vi "test-SwerveDrvPoseEst2-testFollowTrajectory.vi"(0 "chassisSpeedsGenerator":refnum<vi>, 1 "TRAJECTORY":T12 {"States"."POSE"."ROTATION"."SIN" format="%13.4f"; "States"."POSE"."ROTATION"."COS" format="%13.4f"; "States"."POSE"."ROTATION"."VALUE" format="%13.4f"; "States"."POSE"."TRANSLATION"."Y" format="%14.3f"; "States"."POSE"."TRANSLATION"."X" format="%14.3f"; "TotalTImeSecs" format="%20.3f"}, 2 "SwerveDrivePoseEstimate2":T5={"M_Vision_K"=[], "m_nominal_dT"=0.0, "m_PrevTime_Sec"=0.0, "Pose_Buffer"={"TimeStamps"=[], "DataArray"=[], "Min_TimeStamp"=0.0, "Max_TimeStamp"=0.0, "ItemCount"=0, "MaxBufferTime"=0.0}, "Swerve_Drive_Kinematics"={"NumModules"=0, "InverseKinematics"=[], "ForwardKinematics"=[], "Modules"=[], "PrevCoR"={"X"=0.0, "Y"=0.0}, "SavedModuleStates"=[]}, "Swerve_Drive_Odom"={"POSE"={"TRANSLATION"={"X"=0.0, "Y"=0.0}, "ROTATION"={"VALUE"=0.0, "COS"=0.0, "SIN"=0.0}}, "GyroOffset"={"VALUE"=0.0, "COS"=0.0, "SIN"=0.0}, "PreviousAngle"={"VALUE"=0.0, "COS"=0.0, "SIN"=0.0}, "PrevModulePositions"=[], "NumModules"=0}, "M_Q"=[], "NumModules"=-1} {"Swerve_Drive_Odom"."PrevModulePositions"."Angle"."SIN" format="%13.4f"; "Swerve_Drive_Odom"."PrevModulePositions"."Angle"."COS" format="%13.4f"; "Swerve_Drive_Odom"."PrevModulePositions"."Angle"."VALUE" format="%13.4f"; "Swerve_Drive_Odom"."PreviousAngle"."SIN" format="%13.4f"; "Swerve_Drive_Odom"."PreviousAngle"."COS" format="%13.4f"; "Swerve_Drive_Odom"."PreviousAngle"."VALUE" format="%13.4f"; "Swerve_Drive_Odom"."GyroOffset"."SIN" format="%13.4f"; "Swerve_Drive_Odom"."GyroOffset"."COS" format="%13.4f"; "Swerve_Drive_Odom"."GyroOffset"."VALUE" format="%13.4f"; "Swerve_Drive_Odom"."POSE"."ROTATION"."SIN" format="%13.4f"; "Swerve_Drive_Odom"."POSE"."ROTATION"."COS" format="%13.4f"; "Swerve_Drive_Odom"."POSE"."ROTATION"."VALUE" format="%13.4f"; "Swerve_Drive_Odom"."POSE"."TRANSLATION"."Y" format="%14.3f"; "Swerve_Drive_Odom"."POSE"."TRANSLATION"."X" format="%14.3f"; "Swerve_Drive_Kinematics"."SavedModuleStates"."Angle"."SIN" format="%13.4f"; "Swerve_Drive_Kinematics"."SavedModuleStates"."Angle"."COS" format="%13.4f"; "Swerve_Drive_Kinematics"."SavedModuleStates"."Angle"."VALUE" format="%13.4f"; "Swerve_Drive_Kinematics"."PrevCoR"."Y" format="%14.3f"; "Swerve_Drive_Kinematics"."PrevCoR"."X" format="%14.3f"; "Swerve_Drive_Kinematics"."Modules"."Y" format="%14.3f"; "Swerve_Drive_Kinematics"."Modules"."X" format="%14.3f"}, 5 "genVisionMeasurement":refnum<vi>, 7 "StartingPose":T2={"TRANSLATION"={"X"=0.0, "Y"=0.0}, "ROTATION"={"VALUE"=0.0, "COS"=1.0, "SIN"=0.0}} {"ROTATION"."SIN" format="%13.4f"; "ROTATION"."COS" format="%13.4f"; "ROTATION"."VALUE" format="%13.4f"; "TRANSLATION"."Y" format="%14.3f"; "TRANSLATION"."X" format="%14.3f"}, 9 "EndingPose":T2={"TRANSLATION"={"X"=0.0, "Y"=0.0}, "ROTATION"={"VALUE"=0.0, "COS"=1.0, "SIN"=0.0}} {"ROTATION"."SIN" format="%13.4f"; "ROTATION"."COS" format="%13.4f"; "ROTATION"."VALUE" format="%13.4f"; "TRANSLATION"."Y" format="%14.3f"; "TRANSLATION"."X" format="%14.3f"}, 11 "dt_Seconds":dbl, 12 "VisionUpdateRate":dbl, 13 "VisionUpdateDelay":dbl, 14 "CheckError":bool) -> (4 "Test Passed":bool, 6 "Output Data":T1, 15 "DataForGraph":cluster{dbl[], dbl[]}[](array[cluster]))   [LabVIEW 2019]
uses:
  <vilib>/Rock Robotics/WPI/ThirdParty/JAS_Junk/TrajLib/Trajectory_Library.lvlib
  <vilib>/Rock Robotics/WPI/ThirdParty/JAS_Junk/TrajLib/TypeDef/TRANSLATION2D.ctl
  <vilib>/Rock Robotics/WPI/ThirdParty/JAS_Junk/TrajLib/TypeDef/ROTATION2D.ctl
  <vilib>/Rock Robotics/WPI/ThirdParty/JAS_Junk/TrajLib/TypeDef/POSE2D.ctl
  <vilib>/Rock Robotics/WPI/ThirdParty/JAS_Junk/TrajLib/TypeDef/TRAJ_STATE.ctl
  <vilib>/Rock Robotics/WPI/ThirdParty/JAS_Junk/TrajLib/TypeDef/TRAJECTORY.ctl
  <vilib>/Analysis/Matrix/Datatypes/RealMatrix.ctl
  <vilib>/Analysis/Matrix/NI_Matrix.lvlib
  <vilib>/Rock Robotics/WPI/ThirdParty/JAS_Junk/TrajLib/TypeDef/TIME_INTERPOLATABLE_VARIANT.ctl
  <vilib>/Rock Robotics/WPI/ThirdParty/JAS_Junk/TrajLib/TypeDef/SWERVE_DRIVE_MODULE_STATE.ctl
  <vilib>/Rock Robotics/WPI/ThirdParty/JAS_Junk/TrajLib/TypeDef/SWERVE_DRIVE_KINEMATICS.ctl
  <vilib>/Rock Robotics/WPI/ThirdParty/JAS_Junk/TrajLib/TypeDef/SWERVE_DRIVE_MODULE_POSITION.ctl
  <vilib>/Rock Robotics/WPI/ThirdParty/JAS_Junk/TrajLib/TypeDef/SWERVE_DRIVE_ODOMETRY.ctl
  <vilib>/Rock Robotics/WPI/ThirdParty/JAS_Junk/TrajLib/TypeDef/SWERVE_DRIVE_POSE_EST2.ctl
panel:
  in  "UseVIsion":bool=TRUE
  out "error out":errorcluster
  in  "error in (no error)":errorcluster
  # "<3, 1>"
  # "<3, 3>"
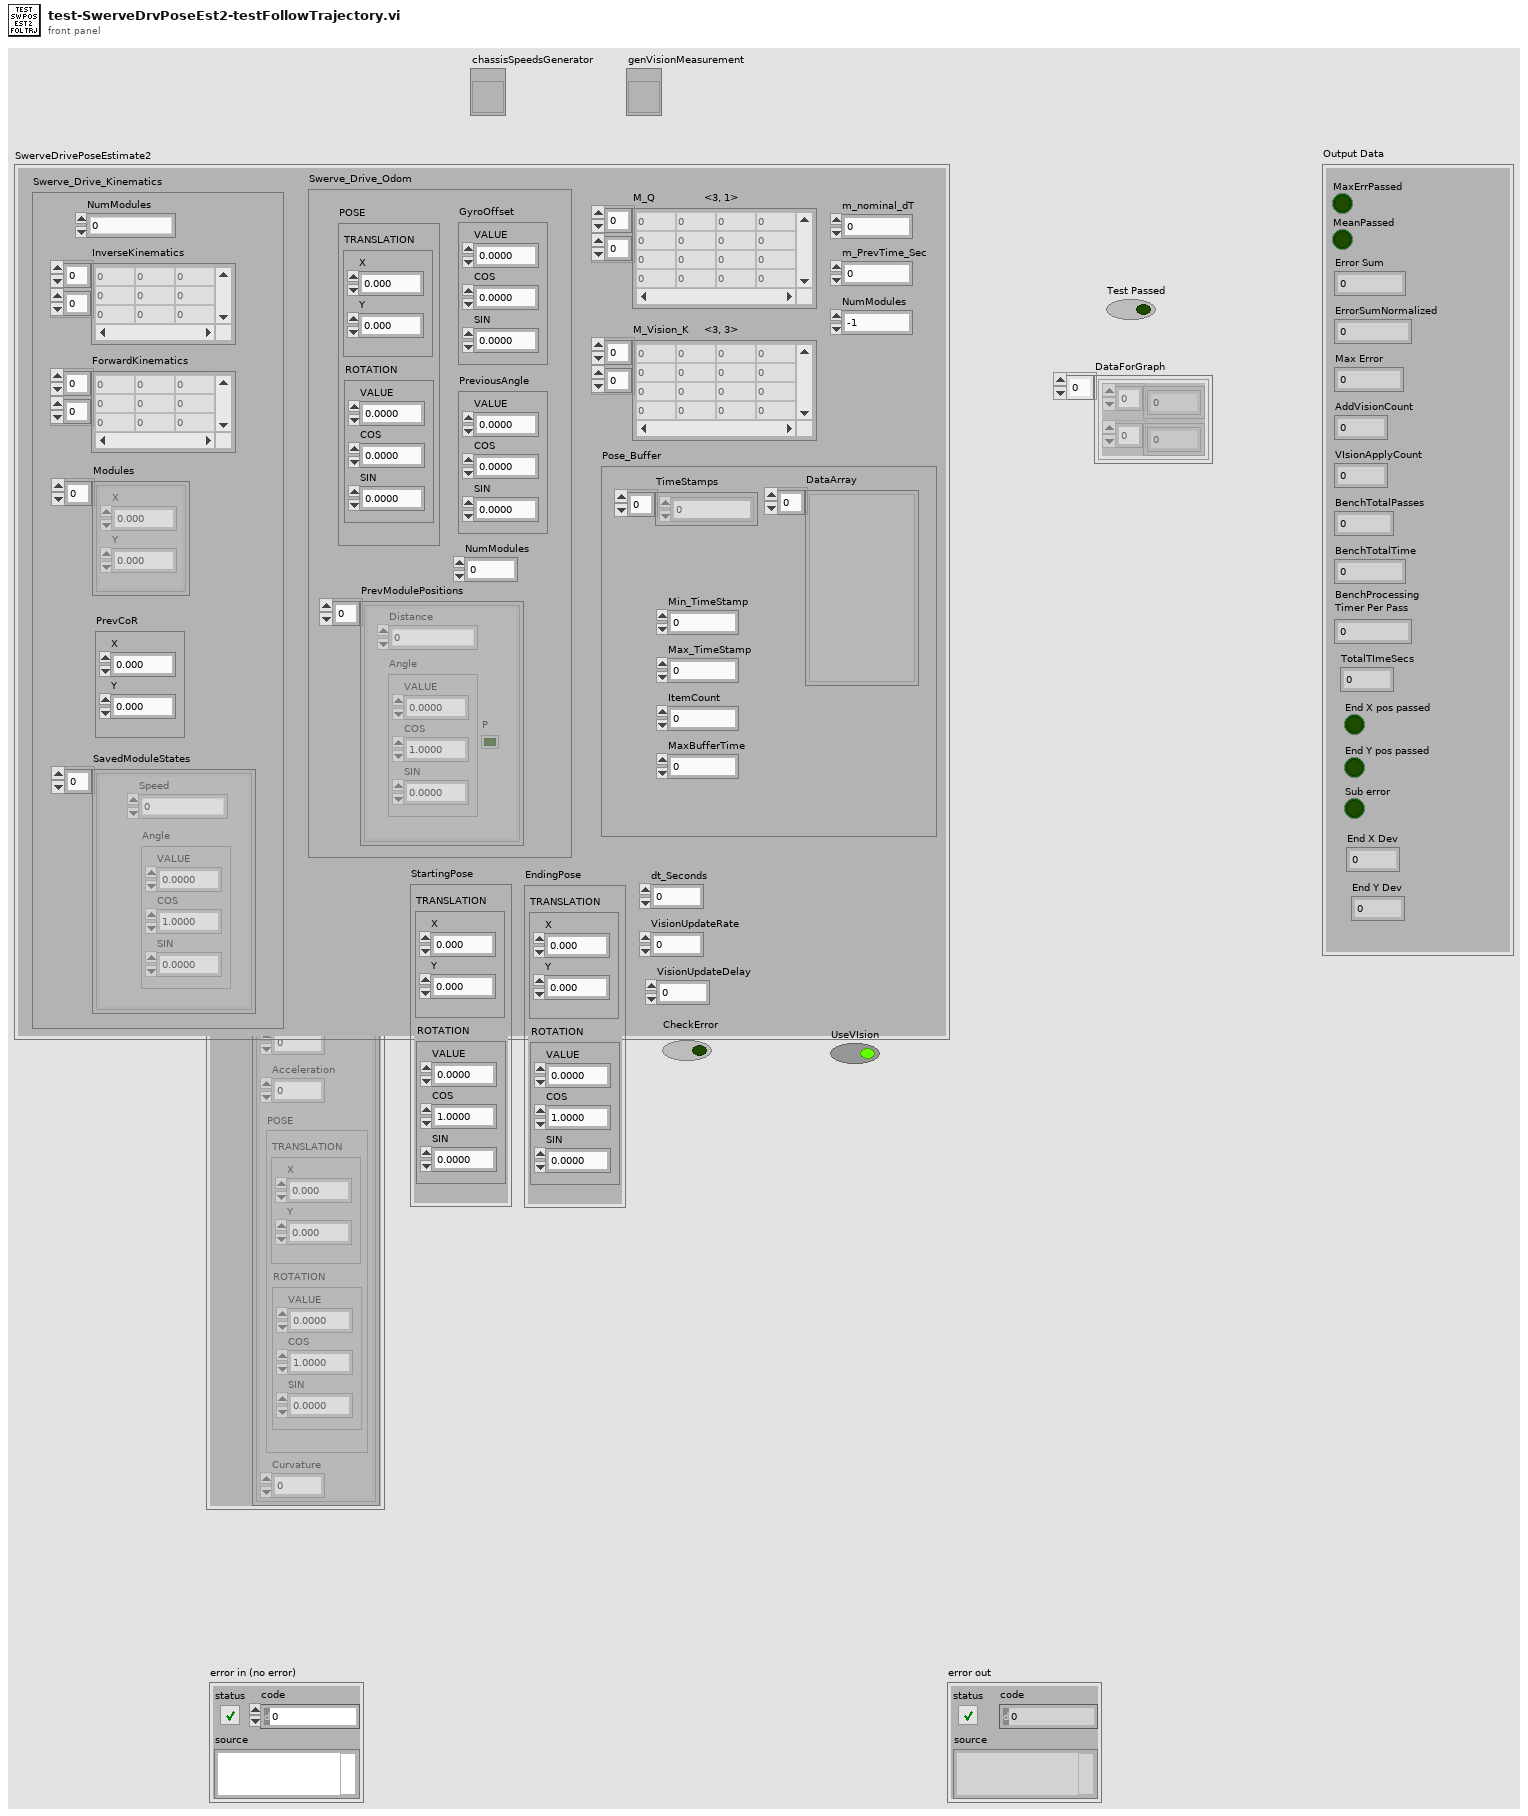
[diagram p1: front panel]
types:
  T1 = cluster{"MaxErrPassed":bool, "MeanPassed":bool, "Error Sum":dbl, "ErrorSumNormalized":dbl, "Max Error":dbl, "AddVisionCount":i32, "VIsionApplyCount":i32, "BenchTotalPasses":dbl, "BenchTotalTime":dbl, "BenchProcessing \nTimer Per Pass":dbl, "TotalTImeSecs":dbl, "End X pos passed":bool, "End Y pos passed":bool, "Sub error":bool, "End X Dev":dbl, "End Y Dev":dbl}
  T2 = typedef "Trajectory_Library.lvlib/POSE2D.ctl" = cluster{"TRANSLATION":T3, "ROTATION":T4}
  T3 = typedef "Trajectory_Library.lvlib/TRANSLATION2D.ctl" = cluster{"X":dbl, "Y":dbl}
  T4 = typedef "Trajectory_Library.lvlib/ROTATION2D.ctl" = cluster{"VALUE":dbl, "COS":dbl, "SIN":dbl}
  T5 = typedef "Trajectory_Library.lvlib/SWERVE_DRIVE_POSE_EST2.ctl" = cluster{"M_Vision_K":T6, "m_nominal_dT":dbl, "m_PrevTime_Sec":dbl, "Pose_Buffer":T7, "Swerve_Drive_Kinematics":T8, "Swerve_Drive_Odom":T10, "M_Q":T6, "NumModules":i32}
  T6 = typedef "NI_Matrix.lvlib/RealMatrix.ctl" = dbl[][]
  T7 = typedef "Trajectory_Library.lvlib/TIME_INTERPOLATABLE_VARIANT.ctl" = cluster{"TimeStamps":dbl[], "DataArray":variant[], "Min_TimeStamp":dbl, "Max_TimeStamp":dbl, "ItemCount":i32, "MaxBufferTime":dbl}
  T8 = typedef "Trajectory_Library.lvlib/SWERVE_DRIVE_KINEMATICS.ctl" = cluster{"NumModules":i32, "InverseKinematics":T6, "ForwardKinematics":T6, "Modules":T3[], "PrevCoR":T3, "SavedModuleStates":T9[]}
  T9 = typedef "Trajectory_Library.lvlib/SWERVE_DRIVE_MODULE_STATE.ctl" = cluster{"Speed":dbl, "Angle":T4}
  T10 = typedef "Trajectory_Library.lvlib/SWERVE_DRIVE_ODOMETRY.ctl" = cluster{"POSE":T2, "GyroOffset":T4, "PreviousAngle":T4, "PrevModulePositions":T11[], "NumModules":i32}
  T11 = typedef "Trajectory_Library.lvlib/SWERVE_DRIVE_MODULE_POSITION.ctl" = cluster{"Distance":dbl, "Angle":T4, "P":bool}
  T12 = typedef "Trajectory_Library.lvlib/TRAJECTORY.ctl" = cluster{"TotalTImeSecs":dbl, "States":T13[]}
  T13 = typedef "Trajectory_Library.lvlib/TRAJ_STATE.ctl" = cluster{"TimeSeconds":dbl, "Velocity":dbl, "Acceleration":dbl, "POSE":T2, "Curvature":dbl}
  T14 = typedef "Trajectory_Library.lvlib/TIME_INTERPOLATABLE_POSE2D.ctl" = cluster{"TimeStamps":dbl[], "Pose":T2[], "Min_TimeStamp":dbl, "Max_TimeStamp":dbl, "ItemCount":i32, "MaxBufferTime":dbl}
  T15 = typedef "Trajectory_Library.lvlib/TRANSFORM2D.ctl" = cluster{"TRANSLATION":T3, "ROTATION":T4, "xF":bool}
  T16 = typedef "Trajectory_Library.lvlib/CHASSIS_SPEEDS.ctl" = cluster{"vX":dbl, "vY":dbl, "vOmega":dbl}
  T17 = cluster{bool, bool, "Error Sum":dbl, dbl, dbl, i32, i32, "TotalPasses":dbl, "TotalTime":dbl, dbl, "TotalTImeSecs":dbl, bool, bool, bool, dbl, dbl}
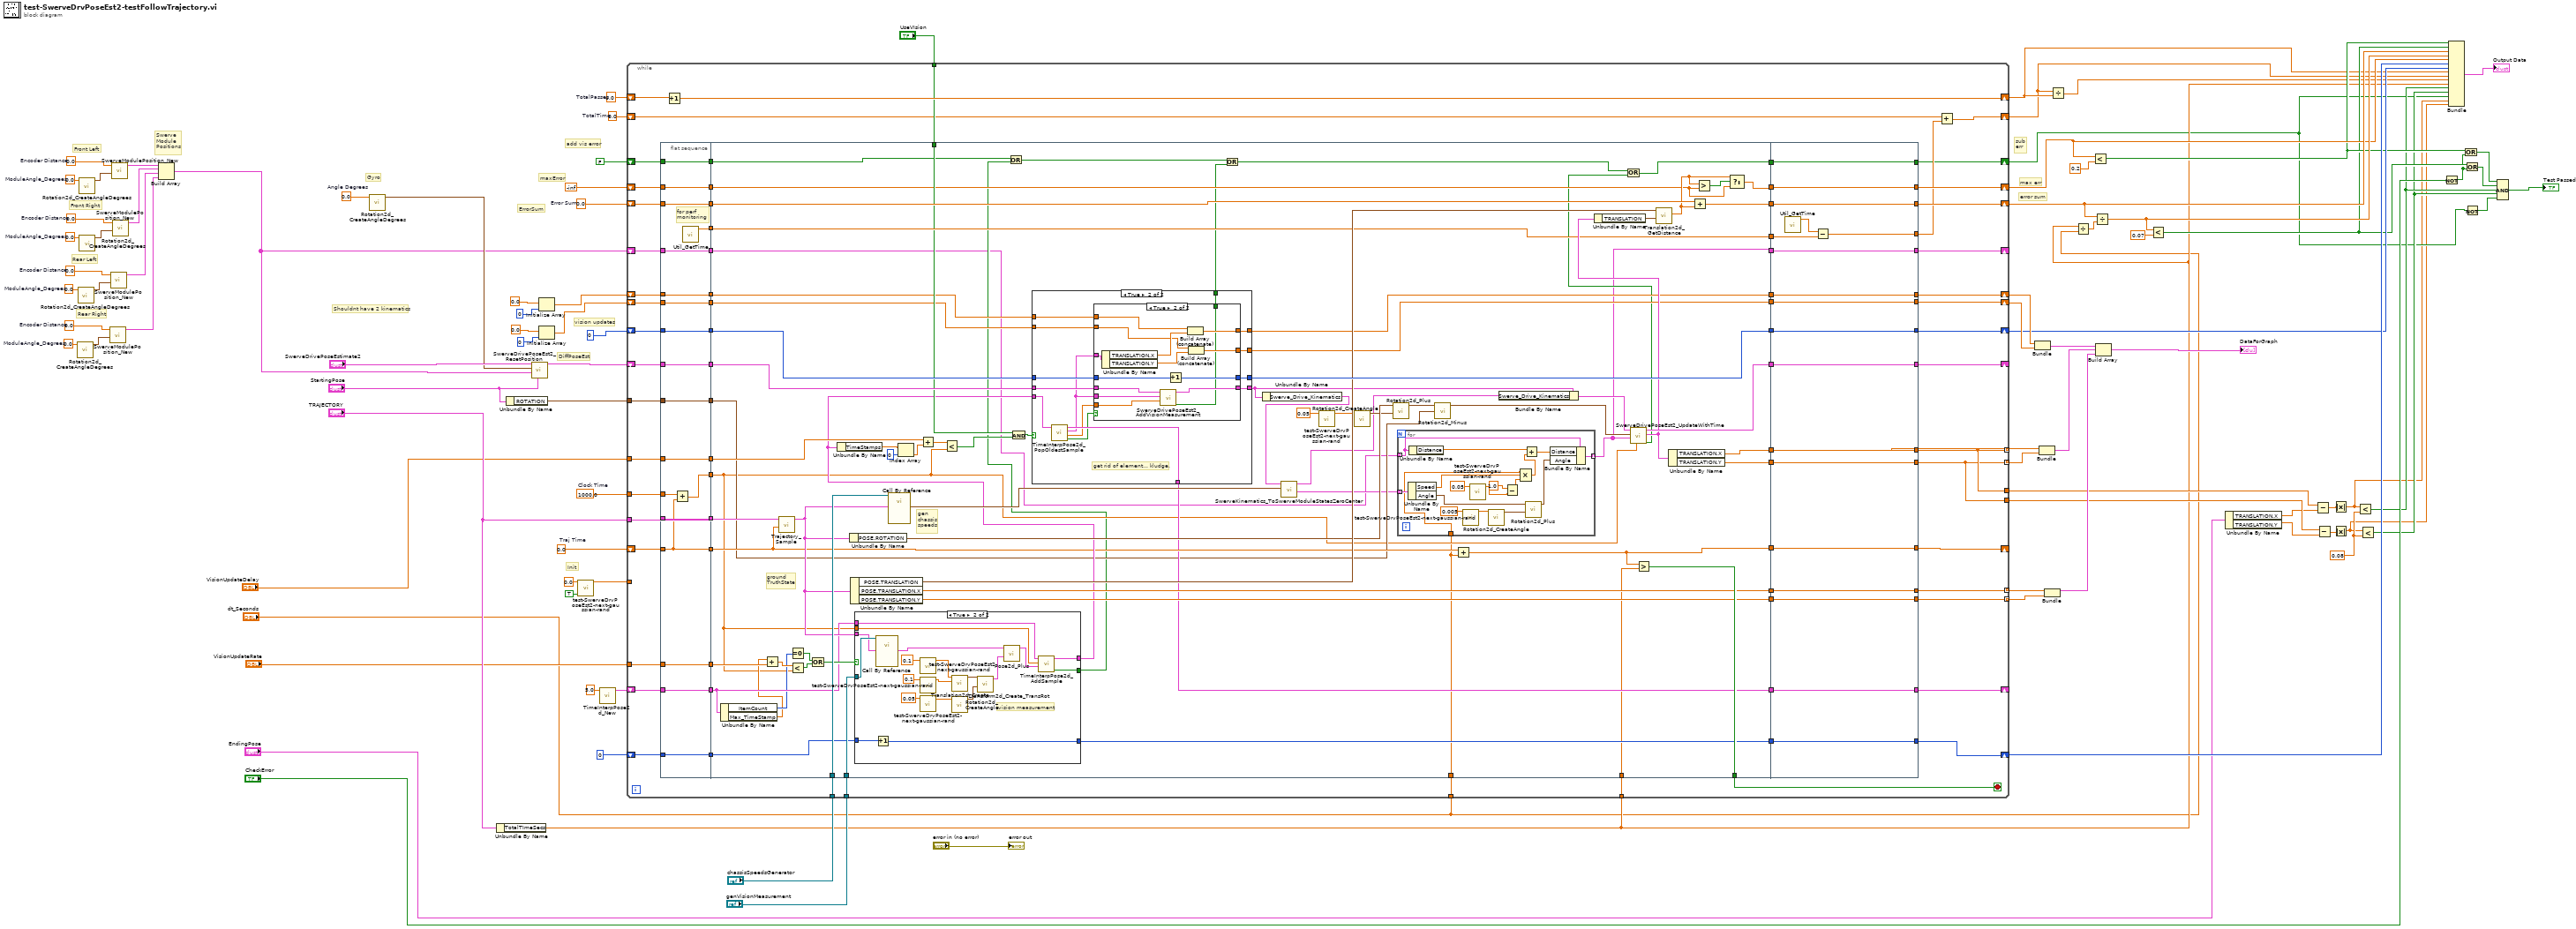
[diagram p0: block diagram]
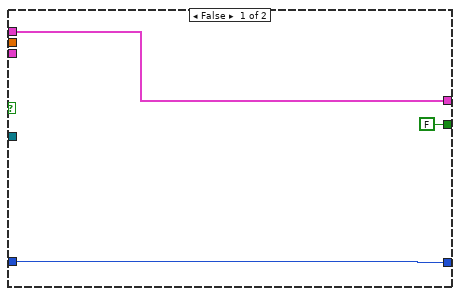
[diagram p2: hidden frame]
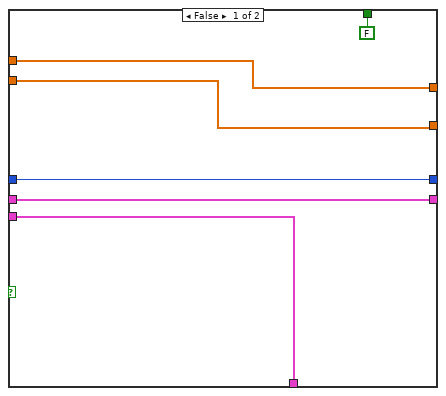
[diagram p3: hidden frame]
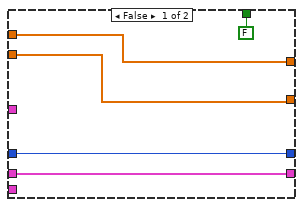
[diagram p4: hidden frame]
diagram:
  w14 = 0.0  # ModuleAngle_Degrees
  w12 = 0.0  # Encoder Distance
  w11 = 0.0  # ModuleAngle_Degrees
  w9 = 0.0  # Encoder Distance
  w8 = 0.0  # ModuleAngle_Degrees
  w6 = 0.0  # Encoder Distance
  w4 = 0.0  # ModuleAngle_Degrees
  w2 = 0.0  # Encoder Distance
  w39 = 0.08
  w64 = 1000.0  # Clock Time
  w72 = 0.0  # Angle Degrees
  w92 = 0.0  # TotalPasses
  w91 = 0.0  # TotalTime
  w86 = 0.0  # Error Sum
  w76 = 0.0  # Traj Time
  # "Shouldnt have 2 kinematics"
  # "Front Left"
  # "Swerve\nModule\nPositions"
  # "Rear Right"
  # "Rear Left"
  # "Front Right"
  # "Init"
  # "sub\nerr"
  # "add vis error"
  # "max err"
  # "error sum"
  # "Gyro"
  # "ErrorSum"
  # "maxError"
  # "vision updates"
  # "DiffPoseEst"
  n1 = call <vilib>:"Rotation2d_CreateAngleDegrees.vi"("Angle_Degrees"=w14) -> ("ROTATION"=w13:T4)  [unwired: 10 in]
  n2 = call <vilib>:"Rotation2d_CreateAngleDegrees.vi"("Angle_Degrees"=w11) -> ("ROTATION"=w10:T4)  [unwired: 10 in]
  n3 = call <vilib>:"Rotation2d_CreateAngleDegrees.vi"("Angle_Degrees"=w4) -> ("ROTATION"=w3:T4)  [unwired: 10 in]
  n4 = call <vilib>:"Rotation2d_CreateAngleDegrees.vi"("Angle_Degrees"=w8) -> ("ROTATION"=w7:T4)  [unwired: 10 in]
  n5 = call <vilib>:"SwerveModulePosition_New.vi"("ROTATION"=w13, "Distance"=w12) -> ("SWERVE_DRIVE_MODULE_POSITION"=w17:T11)  [unwired: 9 in]
  n6 = call <vilib>:"SwerveModulePosition_New.vi"("ROTATION"=w10, "Distance"=w9) -> ("SWERVE_DRIVE_MODULE_POSITION"=w16:T11)  [unwired: 9 in]
  n7 = call <vilib>:"SwerveModulePosition_New.vi"("ROTATION"=w3, "Distance"=w2) -> ("SWERVE_DRIVE_MODULE_POSITION"=w5:T11)  [unwired: 9 in]
  n8 = call <vilib>:"SwerveModulePosition_New.vi"("ROTATION"=w7, "Distance"=w6) -> ("SWERVE_DRIVE_MODULE_POSITION"=w15:T11)  [unwired: 9 in]
  n9 = Build Array(w5, w15, w16, w17) -> (w1:T11[])
  n10 = call <vilib>:"Rotation2d_CreateAngleDegrees.vi"("Angle_Degrees"=w72) -> ("ROTATION"=w71:T4)  [unwired: 10 in]
  n11 = Unbundle By Name("TRAJECTORY") -> ("TotalTImeSecs"=w29:dbl)
  n12 = Unbundle By Name("StartingPose") -> ("ROTATION"=w47:T4)
  n13 = call <vilib>:"SwerveDrivePoseEst2_ResetPosition.vi"("Pose"="StartingPose", "Module Positions"=w1, "Gyro"=w71, "in SwerveDrivePoseEst2"="SwerveDrivePoseEstimate2") -> ("Out SwerveDrivePoseEst2"=w73:T5)  [unwired: 7 in]
  n14 = Initialize Array(0.0, 0 ("dimension size")) -> (w59:dbl[])
  n15 = Initialize Array(0.0, 0 ("dimension size")) -> (w58:dbl[])
  n16 = call "test-SwerveDrvPoseEst2-next-gaussian-rand.vi"("Init"=TRUE, "Multiplier"=0.0 ("R2")) -> ("Gaussian white noise"=w18:dbl)  [unwired: 9 in]
  n17 = call <vilib>:"TimeInterpPose2d_New.vi"("MaxTime"=5.0) -> ("TimeInterpPose"=w68:T14)  [unwired: 10 in]
  n18 = while {
    shift-right: [w170] -> _
    shift-left: w76 -> [w166]
    tunnel: "TRAJECTORY" -> [w168]
    tunnel: w29 -> [w169]
    tunnel: "VisionUpdateRate" -> [w124]
    shift-right: [w135] -> _
    shift-left: w73 -> [w167]
    tunnel: [w106] -> w77 mode=indexing
    tunnel: [w105] -> w78 mode=indexing
    shift-right: [w164] -> w49
    shift-left: 0 -> [w165]
    tunnel: [w163] -> w82 mode=indexing
    tunnel: [w162] -> w83 mode=indexing
    shift-right: [w159] -> w52
    shift-left: -inf -> [w158]
    shift-right: [w160] -> w54
    shift-left: w86 -> [w161]
    shift-right: [w101] -> w31
    shift-left: w91 -> [w102]
    shift-right: [w137] -> w32
    shift-left: w92 -> [w138]
    tunnel: "UseVIsion" -> [w136]
    shift-right: [w132] -> _
    shift-left: w1 -> [w133]
    shift-right: [w127] -> _
    shift-left: w68 -> [w129]
    tunnel: "chassisSpeedsGenerator" -> [w130]
    tunnel: "genVisionMeasurement" -> [w125]
    tunnel: "VisionUpdateDelay" -> [w123]
    tunnel: w64 -> [w121]
    shift-right: [w116] -> w57
    shift-left: w59 -> [w119]
    shift-right: [w114] -> w56
    shift-left: w58 -> [w117]
    shift-right: [w110] -> w50
    shift-left: 0 -> [w111]
    tunnel: w47 -> [w107]
    tunnel: [w106] -> w45
    tunnel: [w105] -> w44
    shift-right: [w98] -> w24
    shift-left: FALSE -> [w99]
    tunnel: "dt_Seconds" -> [w96]
    tunnel: w18 -> [_]
    stop <- w157 stop-if-true
    n19 = flat-sequence {
      tunnel: w158 -> [w183]
      tunnel: w161 -> [w184]
      tunnel: w165 -> [w185]
      tunnel: w166 -> [w177]
      tunnel: w167 -> [w186]
      tunnel: w124 -> [w187]
      tunnel: w168 -> [w188]
      tunnel: [w188] -> w156
      tunnel: [w187] -> w155
      tunnel: [w186] -> w154
      tunnel: [w177] -> w153
      tunnel: [w185] -> w152
      tunnel: [w184] -> w151
      tunnel: [w183] -> w150
      tunnel: [w179] -> w140
      tunnel: [w182] -> w134
      tunnel: w133 -> [w182]
      tunnel: w129 -> [w181]
      tunnel: [w181] -> w128
      tunnel: w123 -> [w180]
      tunnel: [w180] -> w122
      tunnel: w121 -> [w178]
      tunnel: [w176] -> w120
      tunnel: w119 -> [w176]
      tunnel: [w175] -> w118
      tunnel: w117 -> [w175]
      tunnel: [w174] -> w112
      tunnel: w111 -> [w174]
      tunnel: [w173] -> w108
      tunnel: w107 -> [w173]
      tunnel: [w172] -> w104
      tunnel: [w171] -> w100
      tunnel: w99 -> [w171]
      tunnel: [w262] -> w157
      tunnel: w169 -> [w205]
      tunnel: w156 -> [w260]
      tunnel: w155 -> [w232]
      tunnel: w154 -> [w259]
      tunnel: w153 -> [w218]
      tunnel: w152 -> [w255]
      tunnel: w151 -> [w248]
      tunnel: w150 -> [w204]
      tunnel: [w261] -> w149
      tunnel: [w258] -> w148
      tunnel: [w257] -> w147
      tunnel: [w256] -> w146
      tunnel: [w254] -> w145
      tunnel: [w253] -> w144
      tunnel: [w252] -> w143
      tunnel: [w247] -> w142
      tunnel: [w244] -> w141
      tunnel: w140 -> [w243]
      tunnel: [w243] -> w139
      tunnel: w136 -> [w226]
      tunnel: w134 -> [w189]
      tunnel: [w191] -> w131
      tunnel: w130 -> [w239]
      tunnel: w128 -> [w230]
      tunnel: [w217] -> w126
      tunnel: w125 -> [w237]
      tunnel: w122 -> [w223]
      tunnel: w120 -> [w216]
      tunnel: w118 -> [w215]
      tunnel: [w214] -> w115
      tunnel: [w213] -> w113
      tunnel: w112 -> [w212]
      tunnel: [w211] -> w109
      tunnel: w108 -> [w207]
      tunnel: w104 -> [w206]
      tunnel: w100 -> [w199]
      tunnel: [w201] -> w97
      tunnel: w96 -> [w190]
      tunnel: [w350] -> w159
      tunnel: [w351] -> w160
      tunnel: [w352] -> w162
      tunnel: [w353] -> w163
      tunnel: [w354] -> w164
      tunnel: [w355] -> w105
      tunnel: [w356] -> w106
      tunnel: [w357] -> w135
      tunnel: [w358] -> w170
      tunnel: w149 -> [w358]
      tunnel: w148 -> [w357]
      tunnel: w147 -> [w356]
      tunnel: w146 -> [w355]
      tunnel: w145 -> [w354]
      tunnel: w144 -> [w353]
      tunnel: w143 -> [w352]
      tunnel: w142 -> [w351]
      tunnel: w141 -> [w350]
      tunnel: w139 -> [w348]
      tunnel: [w347] -> w132
      tunnel: w131 -> [w347]
      tunnel: [w346] -> w127
      tunnel: w126 -> [w346]
      tunnel: [w345] -> w116
      tunnel: w115 -> [w345]
      tunnel: [w344] -> w114
      tunnel: w113 -> [w344]
      tunnel: [w343] -> w110
      tunnel: w109 -> [w343]
      tunnel: [w342] -> w103
      tunnel: [w341] -> w98
      tunnel: w97 -> [w341]
      frame #0 {
        # "for perf\nmonitoring"
        n20 = Add(x=w178, y=w177) -> (x+y=w172:dbl)
        n21 = call <vilib>:"Util_GetTime.vi"() -> ("FPGA_Time_Seconds"=w179:dbl)  [unwired: 9 in, 2 out]
      }
      frame #1 {
        # "gen\nchassis\nspeeds"
        # "ground\nTruthState"
        n22 = Unbundle By Name(w230) -> ("ItemCount"=w229:i32, "Max_TimeStamp"=w228:dbl)
        n23 = Add(x=w228, y=w232) -> (x+y=w231:dbl)
        n24 = call <vilib>:"Trajectory_Sample.vi"("Time"=w218, "InputTRAJECTORY"=w260) -> ("OutputTRAJ_STATE"=w236:T13)  [unwired: 9 in]
        n25 = Equal To 0?(x=w229) -> (x = 0?=w235:bool)
        n26 = Less?(x=w231, y=w206) -> (x < y?=w234:bool)
        n27 = Compound Arithmetic op=OR(w235, w234) -> (w233:bool)
        n28 = Unbundle By Name(w236) -> ("POSE.ROTATION"=w242:T4)
        n29 = Unbundle By Name(w236) -> ("POSE.TRANSLATION"=w251:T3, "POSE.TRANSLATION.X"=w252:dbl, "POSE.TRANSLATION.Y"=w253:dbl)
        n30 = case shown="True" w233 {
          tunnel: w237 -> [_ w301]
          tunnel: w236 -> [_ w300]
          tunnel: w230 -> [w282 w289]
          tunnel: w206 -> [_ w287]
          tunnel: [w282 w286] -> w220
          tunnel: w212 -> [w281 w285]
          tunnel: [w281 w284] -> w211
          tunnel: [FALSE ("Error") w283] -> w197
          frame False {
          }
          frame True {
            # "vision measurement"
            n31 = Increment(x=w285) -> (x+1=w284:i32)
            n32 = call-by-ref "?"(reference=w301, "TRAJ_STATE"=w300) -> ("POSE2D"=w299:T2)  [unwired: 11 in, 2 out]
            n33 = call "test-SwerveDrvPoseEst2-next-gaussian-rand.vi"("Multiplier"=0.1 ("R0")) -> ("Gaussian white noise"=w294:dbl)  [unwired: 10 in]
            n34 = call "test-SwerveDrvPoseEst2-next-gaussian-rand.vi"("Multiplier"=0.1 ("R1")) -> ("Gaussian white noise"=w295:dbl)  [unwired: 10 in]
            n35 = call "test-SwerveDrvPoseEst2-next-gaussian-rand.vi"("Multiplier"=0.05 ("R2")) -> ("Gaussian white noise"=w296:dbl)  [unwired: 10 in]
            n36 = call <vilib>:"Translation2d_Create.vi"("Y"=w295, "X"=w294) -> ("TRANSLATION"=w297:T3)  [unwired: 9 in]
            n37 = call <vilib>:"Rotation2d_CreateAngle.vi"("Angle"=w296) -> ("ROTATION"=w298:T4)  [unwired: 10 in]
            n38 = call <vilib>:"Transform2d_Create_TransRot.vi"("ROTATION"=w298, "TRANSLATION"=w297) -> ("TRANSFORM"=w290:T15)  [unwired: 9 in]
            n39 = call <vilib>:"Pose2d_Plus.vi"("other TRANSFORM"=w290, "in POSE"=w299) -> ("out POSE"=w288:T2)  [unwired: 9 in]
            n40 = call <vilib>:"TimeInterpPose2d_AddSample.vi"("Pose"=w288, "TimeStamp"=w287, "in TimeInterpPose"=w289) -> ("Error"=w283:bool, "out TimeInterpPose"=w286:T14)  [unwired: 7 in]
          }
        }
        n41 = Unbundle By Name(w220) -> ("TimeStamps"=w225:dbl[])
        n42 = call-by-ref "?"(reference=w239, "TRAJ_STATE"=w236) -> ("CHASSIS"=w238:T16)  [unwired: 11 in, 2 out]
        n43 = Index Array(array=w225, index=0) -> (element=w219:dbl)
        n44 = Add(x=w223, y=w219) -> (x+y=w222:dbl)
        n45 = Less?(x=w222, y=w206) -> (x < y?=w221:bool)
        n46 = Or(x=w199, y=w197) -> (x .or. y?=w198:bool)
        n47 = And(x=w226, y=w221) -> (x .and. y?=w227:bool)
        n48 = case shown="True" w227 {
          tunnel: w259 -> [w307 w321]
          tunnel: [w307 w320] -> w195
          tunnel: w255 -> [w306 w316]
          tunnel: [w306 w315] -> w254
          tunnel: w220 -> [w305 w319]
          tunnel: [w305 w318] -> w217
          tunnel: w216 -> [w304 w312]
          tunnel: w215 -> [w303 w311]
          tunnel: [w304 w310] -> w214
          tunnel: [w303 w309] -> w213
          tunnel: [FALSE ("Error") w308] -> w203
          frame False {
          }
          frame True {
            # "get rid of element... kludge."
            n49 = call <vilib>:"TimeInterpPose2d_PopOldestSample.vi"("in TimeInterpPose2d"=w319) -> ("Is Present"=w317:bool, "TimeStamp"=w314:dbl, "OutputPose2d"=w313:T2, "out TimeInterpPose2d"=w318:T14)  [unwired: 7 in]
            n50 = case shown="True" w317 {
              tunnel: w321 -> [w326 w340]
              tunnel: [w326 w339] -> w320
              tunnel: w316 -> [w325 w338]
              tunnel: [w325 w337] -> w315
              tunnel: w313 -> [_ w336]
              tunnel: w314 -> [_ w335]
              tunnel: w313 -> [_ w334]
              tunnel: w312 -> [w324 w331]
              tunnel: w311 -> [w323 w330]
              tunnel: [w324 w329] -> w310
              tunnel: [w323 w328] -> w309
              tunnel: [FALSE ("Error") w327] -> w308
              frame False {
              }
              frame True {
                n51 = Unbundle By Name(w334) -> ("TRANSLATION.X"=w333:dbl, "TRANSLATION.Y"=w332:dbl)
                n52 = call <vilib>:"SwerveDrivePoseEst2_AddVisionMeasurement.vi"("TImeStamp_Seconds"=w335, "visionRobotPose"=w336, "in SwerveDrivePoseEst2"=w340) -> ("Error"=w327:bool, "Out SwerveDrivePoseEst2"=w339:T5)  [unwired: 7 in]
                n53 = Increment(x=w338) -> (x+1=w337:i32)
                n54 = Build Array (concatenate)(w331, w333) -> (w329:dbl[])
                n55 = Build Array (concatenate)(w330, w332) -> (w328:dbl[])
              }
            }
          }
        }
        n56 = Or(x=w198, y=w203) -> (x .or. y?=w202:bool)
        n57 = Unbundle By Name(w195) -> ("Swerve_Drive_Kinematics"=w196:T8)
        n58 = call <vilib>:"SwerveKinematics_ToSwerveModuleStatesZeroCenter.vi"("ChassisSpeeds"=w238, "in SWERVE_DRIVE_KINEMATICS"=w196) -> ("ModuleStates"=w192:T9[], "out SWERVE_DRIVE_KINEMATICS"=w193:T8)  [unwired: 8 in]
        n59 = call "test-SwerveDrvPoseEst2-next-gaussian-rand.vi"("Multiplier"=0.05 ("R0")) -> ("Gaussian white noise"=w240:dbl)  [unwired: 10 in]
        n60 = call <vilib>:"Rotation2d_CreateAngle.vi"("Angle"=w240) -> ("ROTATION"=w241:T4)  [unwired: 10 in]
        n61 = call <vilib>:"Rotation2d_Plus.vi"("other ROTATION"=w241, "in ROTATION"=w242) -> ("out ROTATION"=w210:T4)  [unwired: 9 in]
        n62 = for {
          tunnel: w192 -> [w279] mode=indexing
          tunnel: w189 -> [w278] mode=indexing
          tunnel: [w277] -> w191 mode=indexing
          tunnel: w190 -> [w265]
          n63 = Unbundle By Name(w279) -> ("Speed"=w264:dbl, "Angle"=w270:T4)
          n64 = Unbundle By Name(w278) -> ("Distance"=w274:dbl)
          n65 = call "test-SwerveDrvPoseEst2-next-gaussian-rand.vi"("Multiplier"=0.005 ("R0")) -> ("Gaussian white noise"=w272:dbl)  [unwired: 10 in]
          n66 = call "test-SwerveDrvPoseEst2-next-gaussian-rand.vi"("Multiplier"=0.05 ("R0")) -> ("Gaussian white noise"=w267:dbl)  [unwired: 10 in]
          n67 = call <vilib>:"Rotation2d_CreateAngle.vi"("Angle"=w272) -> ("ROTATION"=w269:T4)  [unwired: 10 in]
          n68 = Subtract(x=1.0, y=w267) -> (x-y=w263:dbl)
          n69 = Compound Arithmetic op=MULTIPLY(w265, w264, w263) -> (w266:dbl)
          n70 = Add(x=w274, y=w266) -> (x+y=w273:dbl)
          n71 = call <vilib>:"Rotation2d_Plus.vi"("other ROTATION"=w269, "in ROTATION"=w270) -> ("out ROTATION"=w271:T4)  [unwired: 9 in]
          n72 = Bundle By Name(cluster=w278, "Distance"=w273, "Angle"=w271) -> (w277:T11)
        }
        n73 = call <vilib>:"Rotation2d_Minus.vi"("other ROTATION"=w207, "in ROTATION"=w210) -> ("out ROTATION"=w209:T4)  [unwired: 9 in]
        n74 = Add(x=w218, y=w190) -> (x+y=w261:dbl)
        n75 = Bundle By Name(cluster=w195, "Swerve_Drive_Kinematics"=w193) -> (w194:T5)
        n76 = call <vilib>:"SwerveDrivePoseEst2_UpdateWithTime.vi"("CurrentTimeSeconds"=w206, "module Positions"=w191, "GyroAngle"=w209, "in SwerveDrivePoseEst2"=w194) -> ("Error"=w200:bool, "Estimated Pose"=w250:T2, "Out SwerveDrivePoseEst2"=w258:T5)  [unwired: 5 in]
        n77 = Unbundle By Name(w250) -> ("TRANSLATION"=w249:T3)
        n78 = Or(x=w202, y=w200) -> (x .or. y?=w201:bool)
        n79 = Greater?(x=w261, y=w205) -> (0:w262:bool)
        n80 = call <vilib>:"Translation2d_GetDistance.vi"("other Translation"=w249, "In Translation"=w251) -> ("Distance"=w245:dbl)  [unwired: 9 in]
        n81 = Unbundle By Name(w250) -> ("TRANSLATION.X"=w257:dbl, "TRANSLATION.Y"=w256:dbl)
        n82 = Add(x=w248, y=w245) -> (x+y=w247:dbl)
        n83 = Greater?(x=w245, y=w204) -> (0:w246:bool)
        n84 = Select(t=w245, s=w246, f=w204) -> (s? t:f=w244:dbl)
      }
      frame #2 {
        n85 = call <vilib>:"Util_GetTime.vi"() -> ("FPGA_Time_Seconds"=w349:dbl)  [unwired: 9 in, 2 out]
        n86 = Subtract(x=w349, y=w348) -> (x-y=w342:dbl)
      }
    }
    n87 = Increment(x=w138) -> (x+1=w137:dbl)
    n88 = Add(x=w102, y=w103) -> (x+y=w101:dbl)
  }
  n89 = Bundle(w57, w56) -> (w79:cluster{dbl[], dbl[]})  [unwired: 1 in]
  n90 = Bundle(w77, w78) -> (w80:cluster{dbl[], dbl[]})  [unwired: 1 in]
  n91 = Bundle(w83, w82) -> (w84:cluster{dbl[], dbl[]})  [unwired: 1 in]
  n92 = Divide(x=w31, y=w32) -> (x/y=w30:dbl)
  n93 = Divide(x=w29, y="dt_Seconds") -> (x/y=w90:dbl)
  n94 = Less?(x=w52, y=0.2) -> (x < y?=w38:bool)
  n95 = Divide(x=w54, y=w90) -> (x/y=w53:dbl)
  n96 = Build Array(w79, w80, w84) -> (→"DataForGraph":cluster{dbl[], dbl[]}[])
  n97 = Less?(x=w53, y=0.07) -> (x < y?=w37:bool)
  n98 = Unbundle By Name("EndingPose") -> ("TRANSLATION.X"=w43:dbl, "TRANSLATION.Y"=w42:dbl)
  n99 = Subtract(x=w45, y=w43) -> (x-y=w41:dbl)
  n100 = Subtract(x=w44, y=w42) -> (x-y=w40:dbl)
  n101 = Absolute Value(x=w41) -> (abs(x)=w22:dbl)
  n102 = Absolute Value(x=w40) -> (abs(x)=w21:dbl)
  n103 = Less?(x=w22, y=w39) -> (x < y?=w28:bool)
  n104 = Less?(x=w21, y=w39) -> (x < y?=w27:bool)
  n105 = Not(x="CheckError") -> (.not. x?=w36:bool)
  n106 = Bundle(w38, w37, "Error Sum"=w54, w53, w52, w50, w49, "TotalPasses"=w32, "TotalTime"=w31, w30, "TotalTImeSecs"=w29, w28, w27, w24, w22, w21) -> (→"Output Data":T17)  [unwired: 1 in]
  n107 = Or(x=w38, y=w36) -> (x .or. y?=w34:bool)
  n108 = Or(x=w37, y=w36) -> (x .or. y?=w35:bool)
  n109 = Not(x=w24) -> (.not. x?=w25:bool)
  n110 = Compound Arithmetic op=AND(w34, w35, w28, w27, w25) -> (→"Test Passed":bool)
  "error out" <- "error in (no error)"
